vi "Table Scroll.vi"(0 "TableRef":refnum<vi>, 2 "Mode":enum16{"Init", "Settings", "Mouse"}(ring)=enum."Mouse", 5 "Height":cluster{"Max":i32, "Min":i32}, 7 "Width":cluster{"Max":i32, "Min":i32}, 9 "Coords":T1, 11 "HorizScroll":bool, 12 "VertScroll":bool, 13 "Row#s":i32) -> (10 "Scroll Chan":bool, 15 "Scroll Buttons":bool)   [LabVIEW 2019]
uses:
  <vilib>/Utility/miscctls.llb/LVPoint32TypeDef.ctl
  <vilib>/Utility/miscctls.llb/LVPositionTypeDef.ctl
  <vilib>/Utility/miscctls.llb/LVRowAndColumnUnsignedTypeDef.ctl
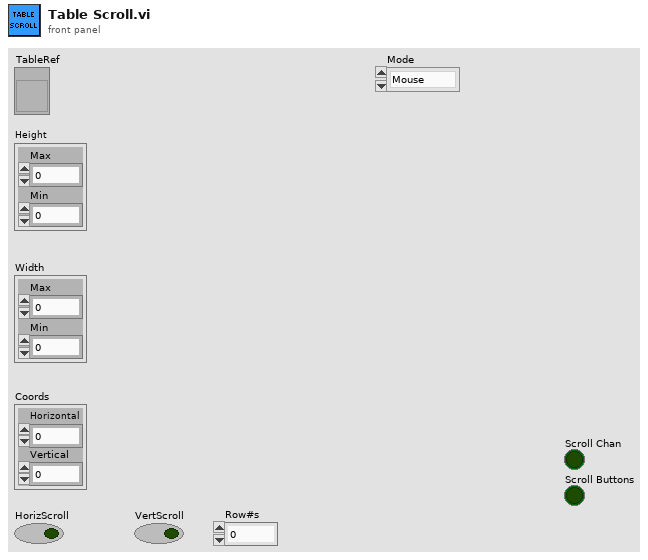
[diagram p1: front panel]
types:
  T1 = typedef "LVPoint32TypeDef.ctl" = cluster{"Horizontal":i32, "Vertical":i32}
  T2 = typedef "LVRowAndColumnUnsignedTypeDef.ctl" = cluster{"Row":u32, "Column":u32}
  T3 = typedef "LVPositionTypeDef.ctl" = cluster{"Left":i32, "Top":i32}
  T4 = cluster{"TableRef":refnum<vi>, "Height":cluster{"Max":i32, "Min":i32}, "Down":cluster{"Max":i32, "Min":i32}, "Up":cluster{"Max":i32, "Min":i32}, "Width":cluster{"Max":i32, "Min":i32}, "Right":cluster{"Max":i32, "Min":i32}, "Left":cluster{"Max":i32, "Min":i32}, "HorizScroll":bool, "VertScroll":bool, "Position":T3, "Row#s":i32}
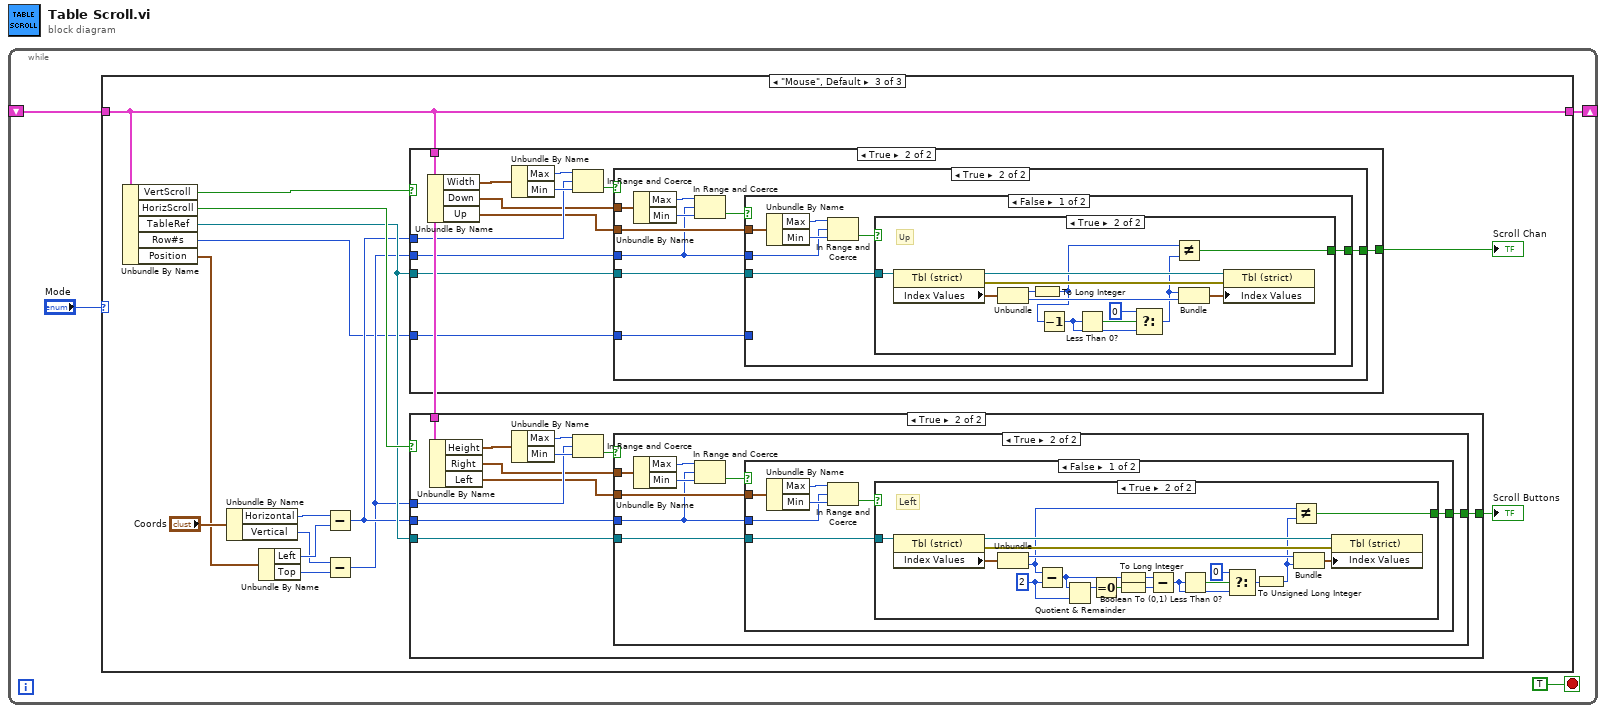
[diagram p0: block diagram]
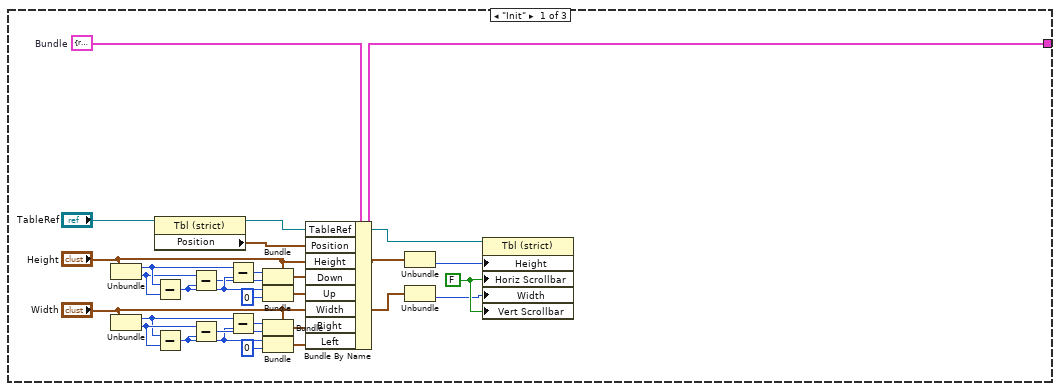
[diagram p2: hidden frame]
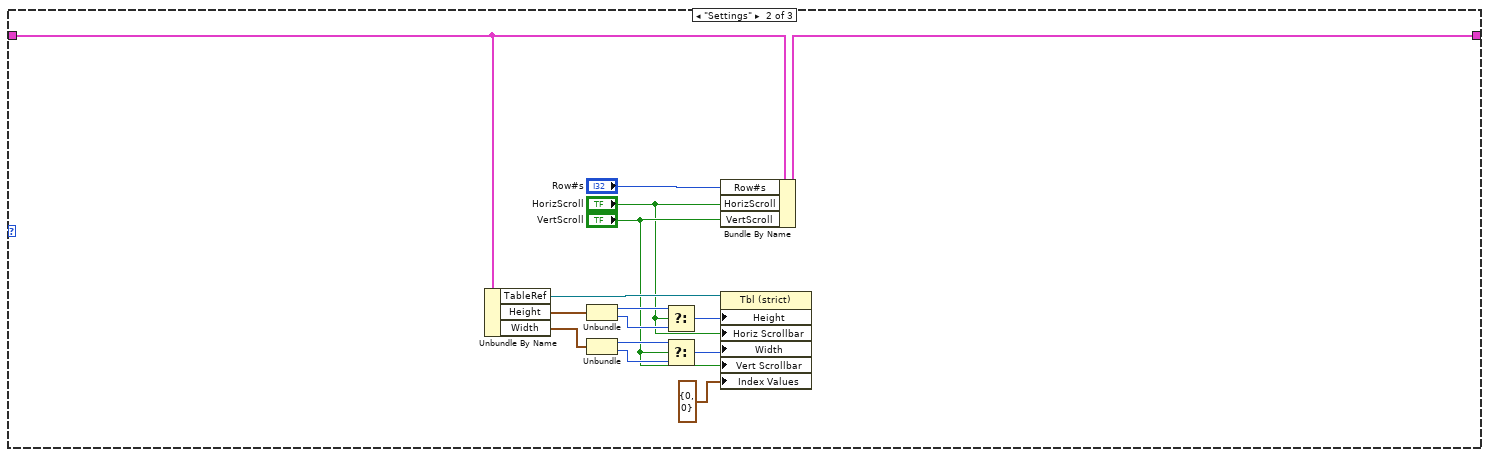
[diagram p3: hidden frame]
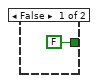
[diagram p4: hidden frame]
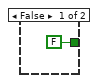
[diagram p5: hidden frame]
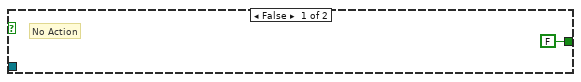
[diagram p6: hidden frame]
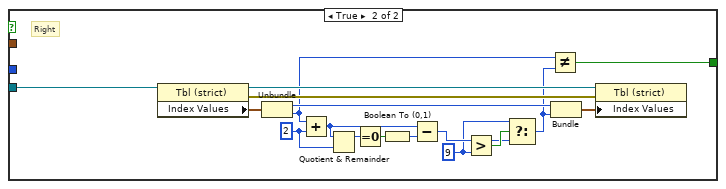
[diagram p7: hidden frame]
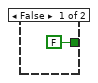
[diagram p8: hidden frame]
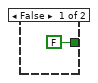
[diagram p9: hidden frame]
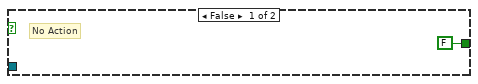
[diagram p10: hidden frame]
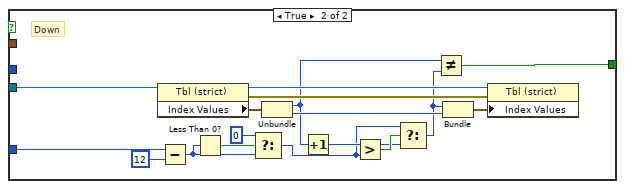
[diagram p11: hidden frame]
diagram:
  n1 = while {
    shift-right: [w2] -> _
    shift-left: _ -> [w1]
    stop <- TRUE stop-if-true
    n2 = case shown="\"Mouse\", Default" "Mode" {
      tunnel: [w30 w45 w54] -> w2
      tunnel: w1 -> [_ w36 w54]
      frame "Init" {
        w5 = T4 {"TableRef"=refnum, "Height"={"Max"=0, "Min"=0}, "Down"={"Max"=0, "Min"=0}, "Up"={"Max"=0, "Min"=0}, "Width"={"Max"=0, "Min"=0}, "Right"={"Max"=0, "Min"=0}, "Left"={"Max"=0, "Min"=0}, "HorizScroll"=FALSE, "VertScroll"=FALSE, "Position"={"Left"=0, "Top"=0}, "Row#s"=0}  # Bundle
        w8 = FALSE
        n3 = Unbundle("Height") -> ("Max"=w19:i32, "Min"=w18:i32)
        n4 = Unbundle("Width") -> ("Max"=w28:i32, "Min"=w29:i32)
        n5 = property class="Tbl (strict)"(reference="TableRef") -> (reference out=w9:refnum<vi>, "Position"=w12:T3)  [unwired: 1 in, 1 out]
        n6 = Subtract(x=w19, y=w18) -> (x-y=w22:i32)
        n7 = Subtract(x=w28, y=w29) -> (x-y=w25:i32)
        n8 = Subtract(x=w18, y=w22) -> (x-y=w21:i32)
        n9 = Subtract(x=w29, y=w25) -> (x-y=w26:i32)
        n10 = Subtract(x=w19, y=w22) -> (x-y=w20:i32)
        n11 = Subtract(x=w28, y=w25) -> (x-y=w27:i32)
        n12 = Bundle(cluster="Height", "Max"=w20, "Min"=w21) -> (w17:cluster{"Max":i32, "Min":i32})
        n13 = Bundle(cluster="Height", "Max"=w22, "Min"=0) -> (w16:cluster{"Max":i32, "Min":i32})
        n14 = Bundle(cluster="Width", "Max"=w27, "Min"=w26) -> (w15:cluster{"Max":i32, "Min":i32})
        n15 = Bundle(cluster="Width", "Max"=w25, "Min"=0) -> (w14:cluster{"Max":i32, "Min":i32})
        n16 = Bundle By Name(cluster=w5, "TableRef"=w9, "Position"=w12, "Height"="Height", "Down"=w17, "Up"=w16, "Width"="Width", "Right"=w15, "Left"=w14) -> (w30:T4)
        n17 = Unbundle("Height") -> ("Min"=w7:i32)  [unwired: 1 out]
        n18 = Unbundle("Width") -> ("Min"=w6:i32)  [unwired: 1 out]
        n19 = property class="Tbl (strict)"(reference=w9, "Height"=w7, "Horiz Scrollbar"=w8, "Width"=w6, "Vert Scrollbar"=w8) -> ()  [unwired: 1 in, 2 out]
      }
      frame "Settings" {
        n20 = Unbundle By Name(w36) -> ("TableRef"=w44:refnum<vi>, "Height"=w43:cluster{"Max":i32, "Min":i32}, "Width"=w38:cluster{"Max":i32, "Min":i32})
        n21 = Unbundle(w43) -> ("Max"=w42:i32, "Min"=w41:i32)
        n22 = Unbundle(w38) -> ("Max"=w39:i32, "Min"=w40:i32)
        n23 = Select(t=w42, s="HorizScroll", f=w41) -> (s? t:f=w37:i32)
        n24 = Select(t=w39, s="VertScroll", f=w40) -> (s? t:f=w35:i32)
        n25 = Bundle By Name(cluster=w36, "Row#s"="Row#s", "HorizScroll"="HorizScroll", "VertScroll"="VertScroll") -> (w45:T4)
        n26 = property class="Tbl (strict)"(reference=w44, "Height"=w37, "Horiz Scrollbar"="HorizScroll", "Width"=w35, "Vert Scrollbar"="VertScroll", "Index Values"=T2 {"Row"=0, "Column"=0}) -> ()  [unwired: 1 in, 2 out]
      }
      frame "Mouse", Default {
        n27 = Unbundle By Name(w54) -> ("VertScroll"=w55:bool, "HorizScroll"=w53:bool, "TableRef"=w52:refnum<vi>, "Row#s"=w48:i32, "Position"=w49:T3)
        n28 = Unbundle By Name("Coords") -> ("Horizontal"=w59:i32, "Vertical"=w57:i32)
        n29 = Unbundle By Name(w49) -> ("Left"=w58:i32, "Top"=w56:i32)
        n30 = Subtract(x=w59, y=w58) -> (x-y=w51:i32)
        n31 = Subtract(x=w57, y=w56) -> (x-y=w50:i32)
        n32 = case shown="True" w55 {
          tunnel: w51 -> [_ w134]
          tunnel: w54 -> [_ w138]
          tunnel: w50 -> [_ w131]
          tunnel: w52 -> [_ w129]
          tunnel: w48 -> [_ w128]
          tunnel: [FALSE w127] -> w47
          frame False {
          }
          frame True {
            n33 = Unbundle By Name(w138) -> ("Width"=w137:cluster{"Max":i32, "Min":i32}, "Down"=w132:cluster{"Max":i32, "Min":i32}, "Up"=w130:cluster{"Max":i32, "Min":i32})
            n34 = Unbundle By Name(w137) -> ("Max"=w136:i32, "Min"=w135:i32)
            n35 = In Range and Coerce(upper limit=w136, x=w134, lower limit=w135) -> (In Range?=w133:bool)  [unwired: 1 out]
            n36 = case shown="True" w133 {
              tunnel: w132 -> [_ w146]
              tunnel: w131 -> [_ w143]
              tunnel: w130 -> [_ w144]
              tunnel: w129 -> [_ w142]
              tunnel: w128 -> [_ w141]
              tunnel: [FALSE w140] -> w127
              frame False {
              }
              frame True {
                n37 = Unbundle By Name(w146) -> ("Max"=w147:i32, "Min"=w148:i32)
                n38 = In Range and Coerce(upper limit=w147, x=w143, lower limit=w148) -> (In Range?=w145:bool)  [unwired: 1 out]
                n39 = case shown="False" w145 {
                  tunnel: w144 -> [w153 _]
                  tunnel: w143 -> [w152 _]
                  tunnel: w142 -> [w150 w180]
                  tunnel: w141 -> [_ w178]
                  tunnel: [w149 w170] -> w140
                  frame False {
                    n40 = Unbundle By Name(w153) -> ("Max"=w155:i32, "Min"=w154:i32)
                    n41 = In Range and Coerce(upper limit=w155, x=w152, lower limit=w154) -> (In Range?=w151:bool)  [unwired: 1 out]
                    n42 = case shown="True" w151 {
                      tunnel: w150 -> [_ w169]
                      tunnel: [FALSE w157] -> w149
                      frame False {
                        # "No Action"
                      }
                      frame True {
                        # "Up"
                        n43 = property class="Tbl (strict)"(reference=w169) -> (reference out=w168:refnum<vi>, error out=w166:errorcluster, "Index Values"=w167:T2)  [unwired: 1 in]
                        n44 = Unbundle(w167) -> ("Row"=w160:u32, "Column"=w164:u32)
                        n45 = To Long Integer(number=w160) -> (32bit integer=w158:i32)
                        n46 = Decrement(x=w158) -> (x-1=w162:i32)
                        n47 = Less Than 0?(x=w162) -> (x < 0?=w163:bool)
                        n48 = Select(t=0, s=w163, f=w162) -> (s? t:f=w159:i32)
                        n49 = Not Equal?(x=w158, y=w159) -> (x != y?=w157:bool)
                        n50 = Bundle("t"=w159, "Column"=w164) -> (w165:cluster{"t":i32, "Column":u32})  [unwired: 1 in]
                        n51 = property class="Tbl (strict)"(reference=w168, error in=w166, "Index Values"=w165) -> ()  [unwired: 2 out]
                      }
                    }
                  }
                  frame True {
                    # "Down"
                    n52 = property class="Tbl (strict)"(reference=w180) -> (reference out=w186:refnum<vi>, error out=w184:errorcluster, "Index Values"=w185:T2)  [unwired: 1 in]
                    n53 = Subtract(x=w178, y=12) -> (x-y=w174:i32)
                    n54 = Less Than 0?(x=w174) -> (x < 0?=w176:bool)
                    n55 = Select(t=0, s=w176, f=w174) -> (s? t:f=w175:i32)
                    n56 = Unbundle(w185) -> ("Row"=w171:u32, "Column"=w182:u32)
                    n57 = Increment(x=w171) -> (x+1=w179:u32)
                    n58 = Greater?(x=w179, y=w175) -> (0:w181:bool)
                    n59 = Select(t=w175, s=w181, f=w179) -> (s? t:f=w172:u32)
                    n60 = Not Equal?(x=w171, y=w172) -> (x != y?=w170:bool)
                    n61 = Bundle("t"=w172, "Column"=w182) -> (w183:cluster{"t":u32, "Column":u32})  [unwired: 1 in]
                    n62 = property class="Tbl (strict)"(reference=w186, error in=w184, "Index Values"=w183) -> ()  [unwired: 2 out]
                  }
                }
              }
            }
          }
        }
        "Scroll Chan" <- w47
        n63 = case shown="True" w53 {
          tunnel: w50 -> [_ w68]
          tunnel: w54 -> [_ w72]
          tunnel: w51 -> [_ w65]
          tunnel: w52 -> [_ w63]
          tunnel: [FALSE w62] -> w46
          frame False {
          }
          frame True {
            n64 = Unbundle By Name(w72) -> ("Height"=w71:cluster{"Max":i32, "Min":i32}, "Right"=w66:cluster{"Max":i32, "Min":i32}, "Left"=w64:cluster{"Max":i32, "Min":i32})
            n65 = Unbundle By Name(w71) -> ("Max"=w70:i32, "Min"=w69:i32)
            n66 = In Range and Coerce(upper limit=w70, x=w68, lower limit=w69) -> (In Range?=w67:bool)  [unwired: 1 out]
            n67 = case shown="True" w67 {
              tunnel: w66 -> [_ w79]
              tunnel: w65 -> [_ w76]
              tunnel: w64 -> [_ w77]
              tunnel: w63 -> [_ w75]
              tunnel: [FALSE w74] -> w62
              frame False {
              }
              frame True {
                n68 = Unbundle By Name(w79) -> ("Max"=w80:i32, "Min"=w81:i32)
                n69 = In Range and Coerce(upper limit=w80, x=w76, lower limit=w81) -> (In Range?=w78:bool)  [unwired: 1 out]
                n70 = case shown="False" w78 {
                  tunnel: w77 -> [w86 _]
                  tunnel: w76 -> [w85 _]
                  tunnel: w75 -> [w83 w114]
                  tunnel: [w82 w109] -> w74
                  frame False {
                    n71 = Unbundle By Name(w86) -> ("Max"=w88:i32, "Min"=w87:i32)
                    n72 = In Range and Coerce(upper limit=w88, x=w85, lower limit=w87) -> (In Range?=w84:bool)  [unwired: 1 out]
                    n73 = case shown="True" w84 {
                      tunnel: w83 -> [_ w108]
                      tunnel: [FALSE w90] -> w82
                      frame False {
                        # "No Action"
                      }
                      frame True {
                        w103 = u32 2 ("y")
                        # "Left"
                        n74 = property class="Tbl (strict)"(reference=w108) -> (reference out=w107:refnum<vi>, error out=w105:errorcluster, "Index Values"=w106:T2)  [unwired: 1 in]
                        n75 = Unbundle(w106) -> ("Row"=w99:u32, "Column"=w91:u32)
                        n76 = Subtract(x=w91, y=w103) -> (x-y=w95:u32)
                        n77 = Quotient & Remainder(x=w95, y=w103) -> (x-y*floor(x/y)=w102:u32)  [unwired: 1 out]
                        n78 = Equal To 0?(x=w102) -> (x = 0?=w101:bool)
                        n79 = To Long Integer(number=w95) -> (32bit integer=w94:i32)
                        n80 = Boolean To (0,1)(Boolean=w101) -> (0, 1=w100:i16)
                        n81 = Subtract(x=w94, y=w100) -> (x-y=w96:i32)
                        n82 = Less Than 0?(x=w96) -> (x < 0?=w98:bool)
                        n83 = Select(t=0, s=w98, f=w96) -> (s? t:f=w93:i32)
                        n84 = To Unsigned Long Integer(number=w93) -> (unsigned 32bit integer=w92:u32)
                        n85 = Not Equal?(x=w91, y=w92) -> (x != y?=w90:bool)
                        n86 = Bundle("Row"=w99, w92) -> (w104:cluster{"Row":u32, u32})  [unwired: 1 in]
                        n87 = property class="Tbl (strict)"(reference=w107, error in=w105, "Index Values"=w104) -> ()  [unwired: 2 out]
                      }
                    }
                  }
                  frame True {
                    w112 = u32 9 ("y")
                    w121 = u32 2 ("y")
                    # "Right"
                    n88 = property class="Tbl (strict)"(reference=w114) -> (reference out=w125:refnum<vi>, error out=w123:errorcluster, "Index Values"=w124:T2)  [unwired: 1 in]
                    n89 = Unbundle(w124) -> ("Row"=w116:u32, "Column"=w110:u32)
                    n90 = Add(x=w110, y=w121) -> (x+y=w118:u32)
                    n91 = Quotient & Remainder(x=w118, y=w121) -> (x-y*floor(x/y)=w120:u32)  [unwired: 1 out]
                    n92 = Equal To 0?(x=w120) -> (x = 0?=w119:bool)
                    n93 = Boolean To (0,1)(Boolean=w119) -> (0, 1=w117:i16)
                    n94 = Subtract(x=w118, y=w117) -> (x-y=w113:u32)
                    n95 = Greater?(x=w113, y=w112) -> (0:w115:bool)
                    n96 = Select(t=w112, s=w115, f=w113) -> (s? t:f=w111:u32)
                    n97 = Not Equal?(x=w110, y=w111) -> (x != y?=w109:bool)
                    n98 = Bundle("Row"=w116, "y"=w111) -> (w122:cluster{"Row":u32, "y":u32})  [unwired: 1 in]
                    n99 = property class="Tbl (strict)"(reference=w125, error in=w123, "Index Values"=w122) -> ()  [unwired: 2 out]
                  }
                }
              }
            }
          }
        }
        "Scroll Buttons" <- w46
      }
    }
  }
